vi "ep_Operate Calibration Instrument.vi"(0 "frequency [Hz]":dbl=50.0, 1 "output state (F: OFF)":bool, 2 "harmonics state (F: OFF)":bool, 5 "voltage RMS [V]":dbl=230.0, 7 "current RMS [A]":dbl=1.0, 9 "harmonics":T1={"harmonic"=3, "voltage amplitude [%]"=10.0, "voltage phase [°]"=0.0, "current amplitude [%]"=10.0, "current phase [°]"=0.0}, 11 "error in (no error)":errorcluster) -> (15 "error out":errorcluster)   [LabVIEW 2012]
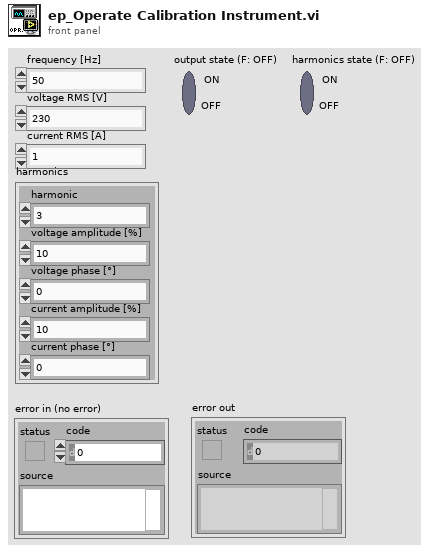
[diagram p1: front panel]
types:
  T1 = cluster{"harmonic":u32, "voltage amplitude [%]":dbl, "voltage phase [°]":dbl, "current amplitude [%]":dbl, "current phase [°]":dbl}
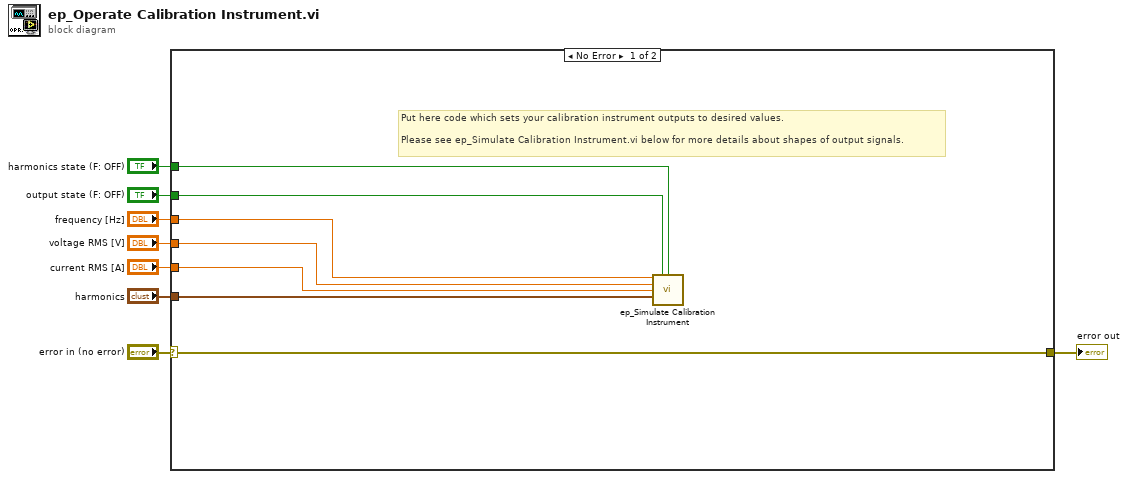
[diagram p0: block diagram]
diagram:
  n1 = case shown="No Error" "error in (no error)" {
    selector: "error in (no error)" -> [w15 w16]
    tunnel: [w15 w16] -> w6
    tunnel: "frequency [Hz]" -> [w12 _]
    tunnel: "voltage RMS [V]" -> [w11 _]
    tunnel: "current RMS [A]" -> [w10 _]
    tunnel: "output state (F: OFF)" -> [w13 _]
    tunnel: "harmonics" -> [w9 _]
    tunnel: "harmonics state (F: OFF)" -> [w14 _]
    frame No Error {
      # "Put here code which sets your calibration instrument outputs to desired values.\n\nPlease see ep_Simulate Calibration Instrument.vi below for more details about shapes of output signals."
      n2 = call <vilib>:"ep_Simulate Calibration Instrument.vi"("frequency [Hz]"=w12, "output state (F: OFF)"=w13, "harmonics state (F: OFF)"=w14, "voltage RMS [V]"=w11, "current RMS [A]"=w10, "harmonics"=w9) -> ()  [unwired: 8 in, 2 out]
    }
    frame Error {
    }
  }
  "error out" <- w6
